vi "getSubArray1D.vi"(8 "error in (no error)":errorcluster, 9 "Index Array Cluster":cluster{"Idx of Dim 0":i32[]}, 10 "1D Array":dbl[](array[numeric]), 11 "MatOper in":refnum<class "MatOper.lvclass">) -> (0 "error out":errorcluster, 2 "Sub-Array":dbl[](array[numeric]), 3 "MatOper out":refnum<class "MatOper.lvclass">)   [LabVIEW 2016, in "OfcFunc.lvlib" / "MatOper.lvclass"]
doc: "Get the sub-array of the specific 1D array based on the index array."
uses:
  MatOper.lvclass
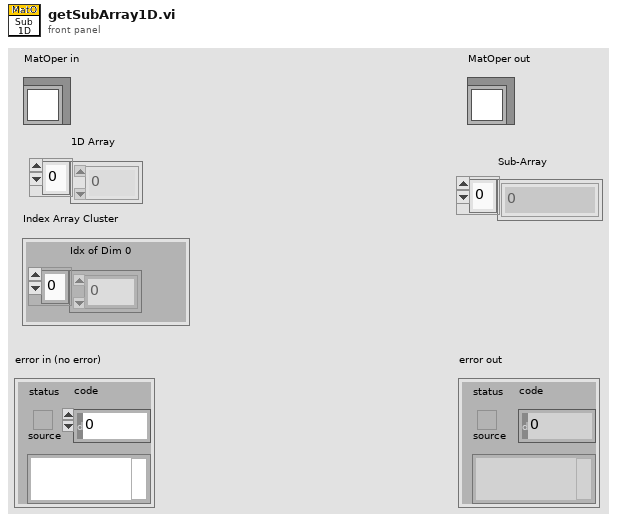
[diagram p1: front panel]
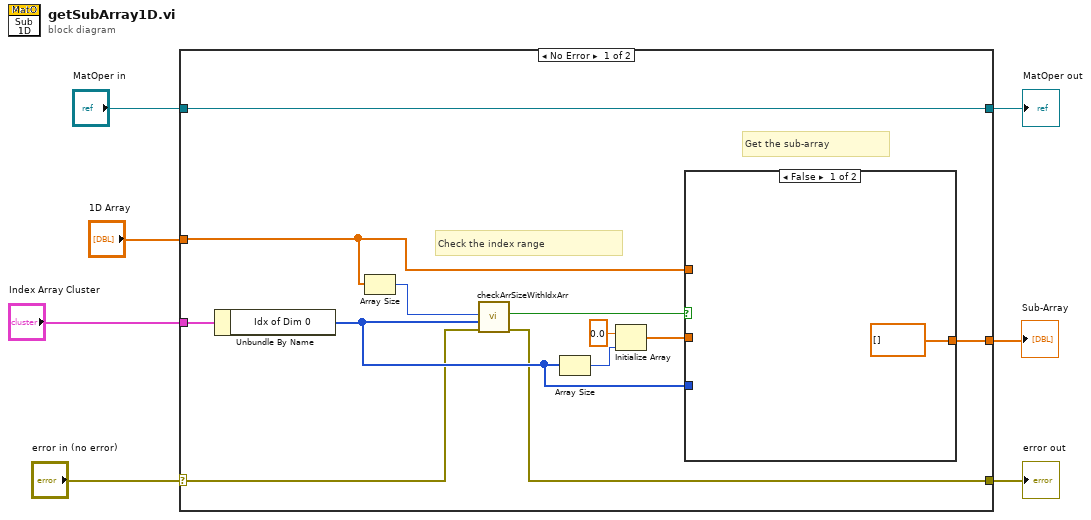
[diagram p0: block diagram]
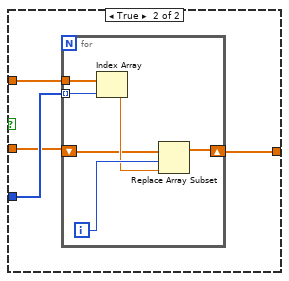
[diagram p2: hidden frame]
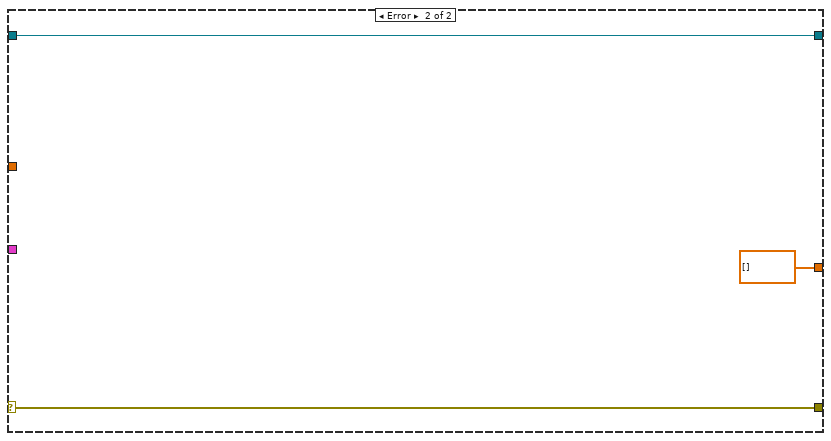
[diagram p3: hidden frame]
diagram:
  n1 = case shown="No Error" "error in (no error)" {
    selector: "error in (no error)" -> [w9 w33]
    tunnel: [w8 w33] -> w6
    tunnel: [w10 w32] -> w4
    tunnel: "MatOper in" -> [w10 w32]
    tunnel: [w16 dbl[] []] -> w3
    tunnel: "Index Array Cluster" -> [w15 _]
    tunnel: "1D Array" -> [w14 _]
    frame No Error {
      # "Get the sub-array"
      # "Check the index range"
      n2 = Unbundle By Name(w15) -> ("Idx of Dim 0"=w11:i32[])
      n3 = Array Size(array=w14) -> (size(s)=w12:i32)
      n4 = call "checkArrSizeWithIdxArr.vi"("error in (no error)"=w9, "Idx Array"=w11, "Array Size"=w12) -> ("error out"=w8:errorcluster, "In Spec"=w13:bool)  [unwired: 6 in, 1 out]
      n5 = Array Size(array=w11) -> (size(s)=w18:i32)
      n6 = Initialize Array(0.0 ("element"), w18) -> (w17:dbl[])
      n7 = case shown="False" w13 {
        tunnel: w14 -> [_ w24]
        tunnel: w11 -> [_ w23]
        tunnel: w17 -> [_ w22]
        tunnel: [dbl[] [] w21] -> w16
        frame False {
        }
        frame True {
          n8 = for {
            tunnel: w24 -> [w30]
            tunnel: w23 -> [w29] mode=indexing
            shift-right: [w25] -> w21
            shift-left: w22 -> [w26]
            i -> [w28]
            n9 = Index Array(array=w30, index=w29) -> (element=w27:dbl)
            n10 = Replace Array Subset(array=w26, new element=w27, index=w28) -> (w25:dbl[])
          }
        }
      }
    }
    frame Error {
    }
  }
  "error out" <- w6
  "MatOper out" <- w4
  "Sub-Array" <- w3
